vi "Position_Config.vi"(8 "error in (no error)":errorcluster, 10 "Position Config":T1, 11 "Step":enum16{"Initial", "Write", "Read"}(ring)) -> (0 "error out":errorcluster, 3 "Position Config out":T1)   [LabVIEW 2017]
uses:
  Ctrls/Position Config.ctl
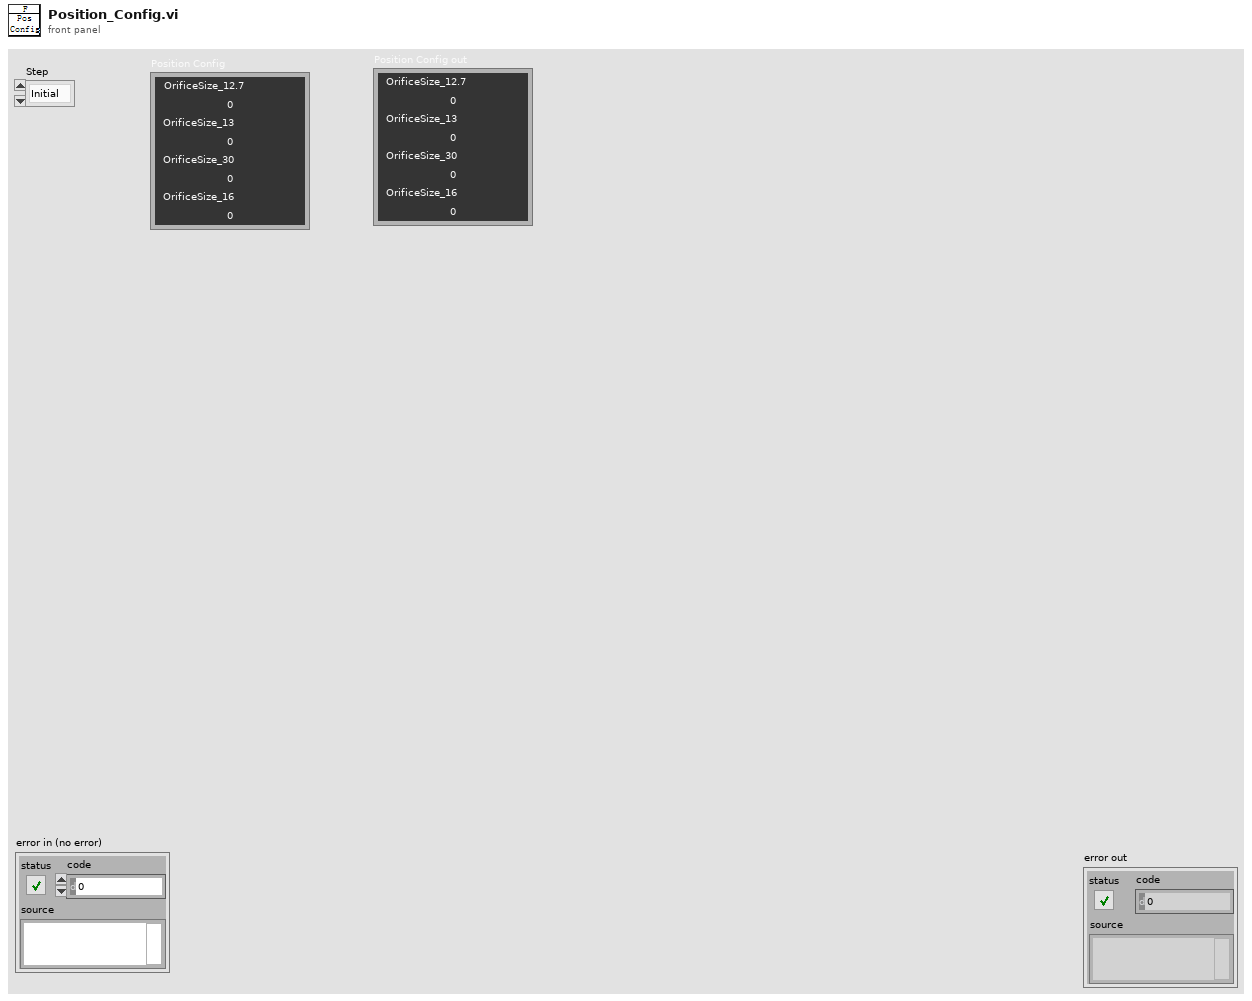
[diagram p1: front panel]
types:
  T1 = typedef "Position Config.ctl" = cluster{"OrificeSize_12.7":i32, "OrificeSize_13":i32, "OrificeSize_30":i32, "OrificeSize_16":i32}
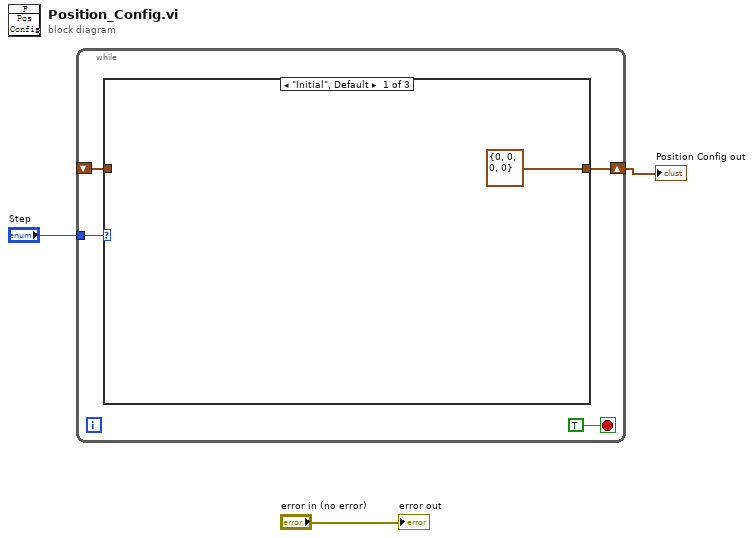
[diagram p0: block diagram]
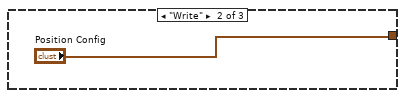
[diagram p2: hidden frame]
diagram:
  n1 = while {
    tunnel: "Step" -> [w6]
    shift-right: [w5] -> w1
    shift-left: _ -> [w4]
    stop <- TRUE stop-if-true
    n2 = case shown="\"Initial\", Default" w6 {
      tunnel: [T1 {"OrificeSize_12.7"=0, "OrificeSize_13"=0, "OrificeSize_30"=0, "OrificeSize_16"=0} ("Position Config") "Position Config" w10] -> w5
      tunnel: w4 -> [_ _ w10]
      frame "Initial", Default {
      }
      frame "Write" {
      }
      frame "Read" {
      }
    }
  }
  "Position Config out" <- w1
  "error out" <- "error in (no error)"
